vi "Configure Measurement Range.vi"(6 "Manual Range (1.0)":dbl=1.0, 8 "error in (no error)":errorcluster, 9 "Enable Auto Range (T:Enable)":bool=TRUE, 10 "Function (0: Volts)":u16(ring) items=["Volts", "Current", "Resistance"], 11 "VISA resource name":refnum<visa-resource-name>) -> (0 "error out":errorcluster, 3 "VISA resource name out":refnum<visa-resource-name>)   [LabVIEW 2022 SP3, in "Keithley 2450.lvlib"]
doc: "Configures the measurement type, resolution, and range on the instrument.\n\n<B>Note:</B> This VI should be called for each measurement that is of interest. This VI can be called multiple times in a row."
uses:
  Keithley 2450.lvlib
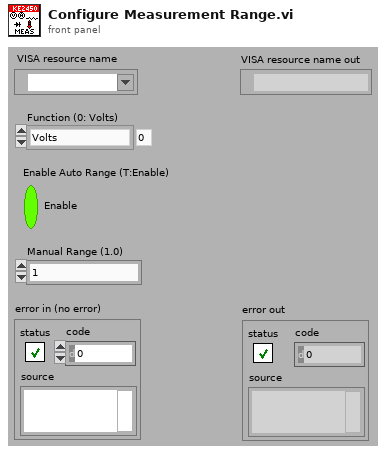
[diagram p1: front panel]
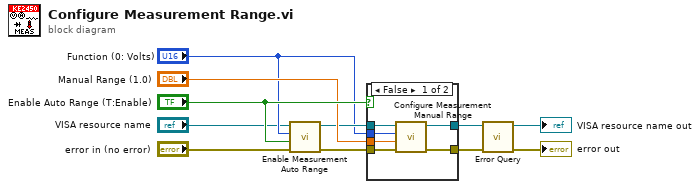
[diagram p0: block diagram]
diagram:
  n1 = call "Enable Measurement Auto Range.vi"("error in (no error)"="error in (no error)", "Enable Auto Range (T:Enable)"="Enable Auto Range (T:Enable)", "Function (0: Volts)"="Function (0: Volts)", "VISA resource name"="VISA resource name") -> ("error out"=w6:errorcluster, "VISA resource name out"=w7:refnum<visa-resource-name>)  [unwired: 6 in]
  n2 = case shown="False" "Enable Auto Range (T:Enable)" {
    tunnel: w7 -> [w17 w19]
    tunnel: "Manual Range (1.0)" -> [w13 _]
    tunnel: w6 -> [w16 w18]
    tunnel: [w15 w19] -> w5
    tunnel: [w14 w18] -> w4
    tunnel: "Function (0: Volts)" -> [w12 _]
    frame False {
      n3 = call "Configure Measurement Manual Range.vi"("error in (no error)"=w16, "Manual Range (1.0)"=w13, "Function (0: Volts)"=w12, "VISA resource name"=w17) -> ("error out"=w14:errorcluster, "VISA resource name out"=w15:refnum<visa-resource-name>)  [unwired: 6 in]
    }
    frame True {
    }
  }
  n4 = call "Error Query.vi"("error in (no error)"=w4, "VISA resource name"=w5) -> ("error out"=→"error out":errorcluster, "VISA resource name out"=→"VISA resource name out":refnum<visa-resource-name>)  [unwired: 8 out]
